vi "Test CD Mgr API.vi"() -> ()   [LabVIEW 2015]
doc: "Probe Mgr API Tester."
uses:
  Collect Data Mgr.lvlib
  Data Collect Parameters typedef--cluster.ctl
  Tool Module/Tool Module.lvlib
  Tool Config/Tool Cfg.lvlib
  Tool Interface/Tool Interface.lvlib
  Tool Interface/_Host - HS Data Stream State Enum Typedef.ctl
  Tool Typedefs/_Data Stream Fmt Params Cluster--typedef.ctl
  Start Collect (Reply Payload)--cluster.ctl
  Stop Collect (Reply Payload)--cluster.ctl
panel:
  in  "data value reference":refnum<data-value>
  out "All Stop":bool
  out "latest notification":u32[](array[numeric])
  out "Position Plot":i32[](graph)
  out "Fault":u8
  out "Position":i32
  in  "Move to Scan Start":bool
  out "Fault or Limit?":bool
  out "At Home?":bool
  in  "Check Home":bool
  in  "Home":bool
  out "Connected":bool
  out "Reply Payload":T1
  in  "Stop Collect":bool
  out "Start Collect (Reply Payload)":T2
  in  "Start Collect":bool
  in  "Show Block Diagram":bool
  in  "Stop Module":bool
  in  "Start Module":bool
  in  "Hide Module Panel":bool
  in  "Show Module Panel":bool
  out "Status":string
  out "Module Running?":bool
  # "This VI tests the API for the Module."
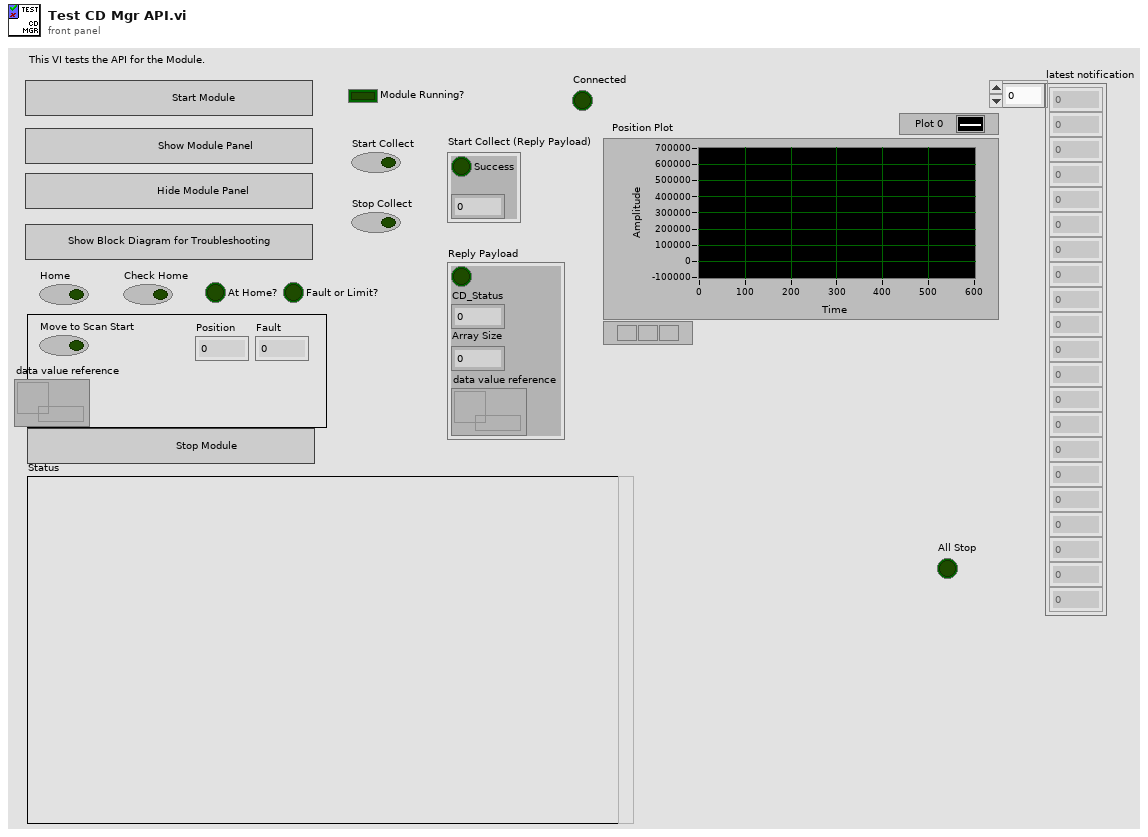
[diagram p1: front panel]
types:
  T1 = typedef "Collect Data Mgr.lvlib/Stop Collect (Reply Payload)--cluster.ctl" = cluster{"Success":bool, "CD_Status":i32, "Array Size":u32, "data value reference":refnum<data-value>}
  T2 = typedef "Collect Data Mgr.lvlib/Start Collect (Reply Payload)--cluster.ctl" = cluster{"Success":bool, "CD_Status":u8}
  T3 = typedef "Tool Interface.lvlib/_Host - HS Data Stream State Enum Typedef.ctl" = enum16{"Idle", "Connect", "Receive Data", "Close Connection"}
  T4 = typedef "Tool Interface.lvlib/_Host - HS Data Stream State Enum Typedef.ctl" = enum16{"Idle", "Connect", "Receive HS Data", "Close Connection"}
  T5 = typedef "Tool Cfg.lvlib/_Tool Operation Config Cluster--typedef.ctl" = cluster{"Use Tool Cfg":bool, "Use Tool Cal":bool, "Fake Data?":bool, "Mode":i16, "Array Subset Length":i16, "nArrays to Read":i16, "Full Array Read Length":i16, "nSubarrays/Sensor":i16}
  T6 = typedef "Collect Data Mgr.lvlib/Broadcast Events--cluster.ctl" = cluster{"Module Did Init":refnum<user-event>, "Status Updated":refnum<user-event>, "Error Reported":refnum<user-event>, "Module Did Stop":refnum<user-event>, "Update Module Execution Status":refnum<user-event>}
  T7 = typedef "_Data Stream Fmt Params Cluster--typedef.ctl" = cluster{"Samples per Block":i32, "Raw Data Status Len":i32, "Fltr Data Status Len":i32}
  T8 = typedef "Collect Data Mgr.lvlib/Data Collect Parameters typedef--cluster.ctl" = cluster{"Mode":i8, "Move Length":i32, "Array Length":i32, "Max Samples":i32}
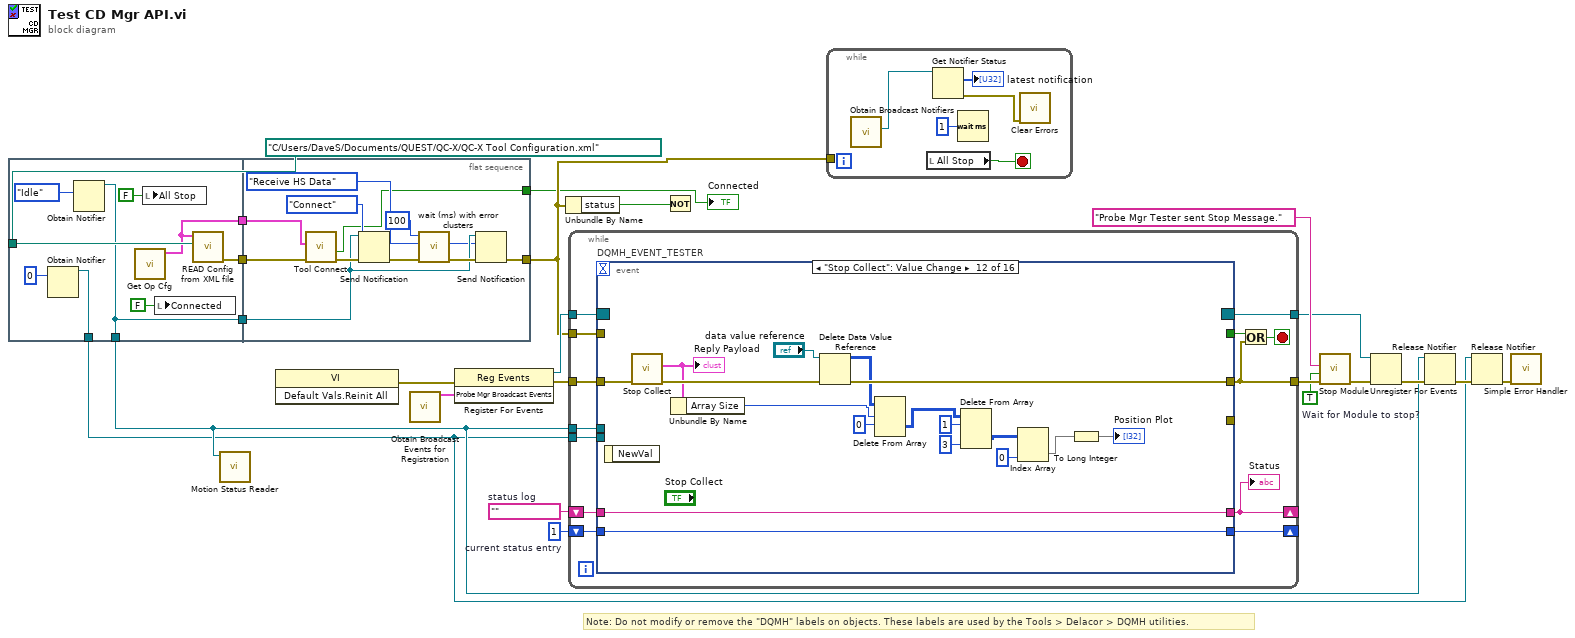
[diagram p0: block diagram]
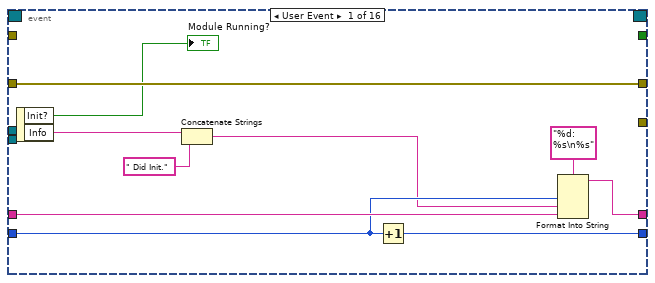
[diagram p2: hidden frame]
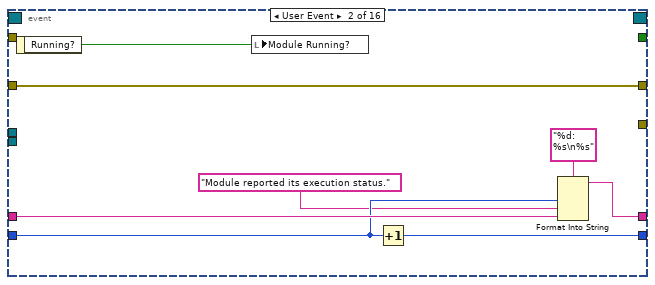
[diagram p3: hidden frame]
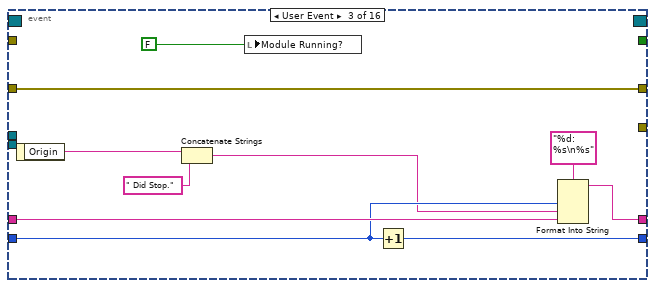
[diagram p4: hidden frame]
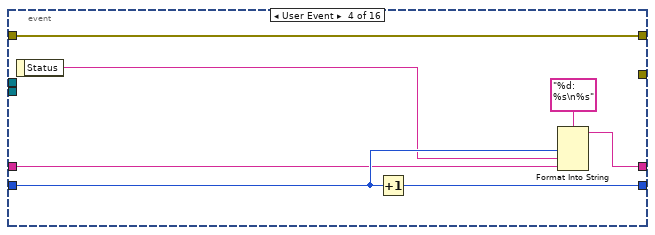
[diagram p5: hidden frame]
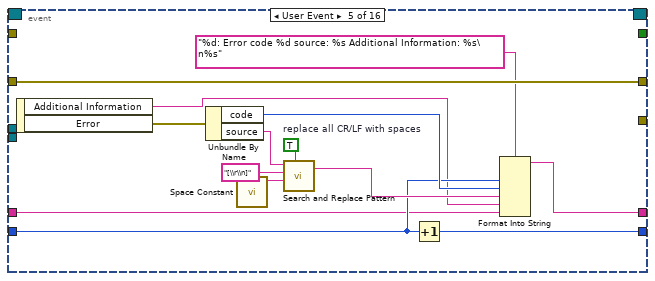
[diagram p6: hidden frame]
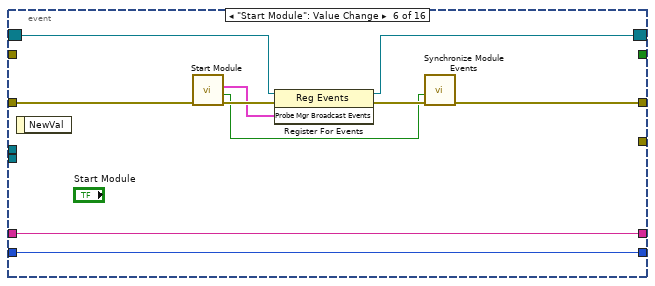
[diagram p7: hidden frame]
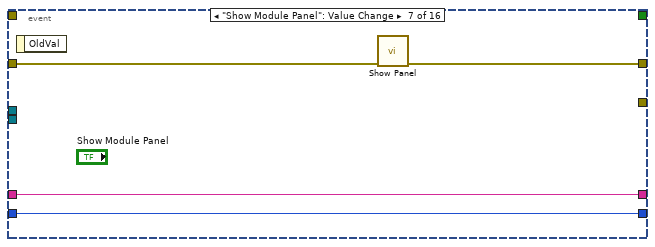
[diagram p8: hidden frame]
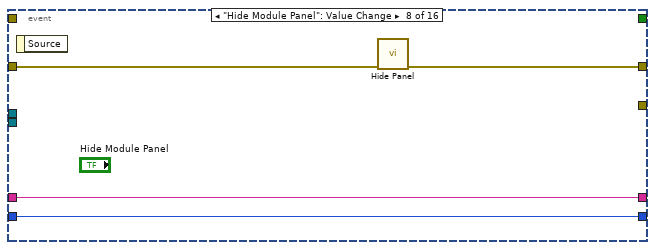
[diagram p9: hidden frame]
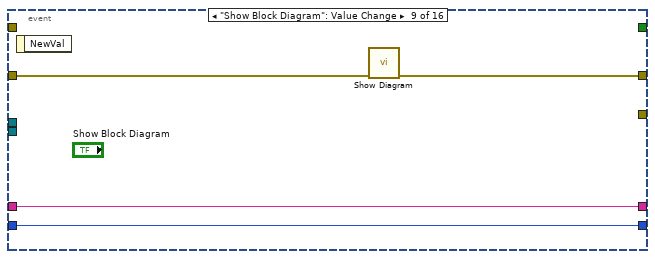
[diagram p10: hidden frame]
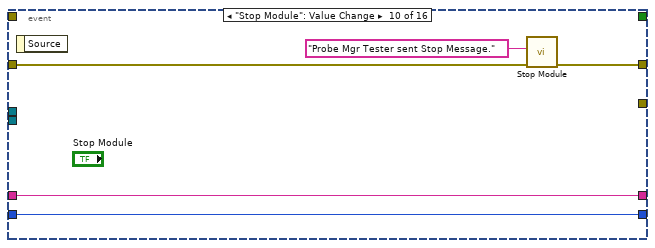
[diagram p11: hidden frame]
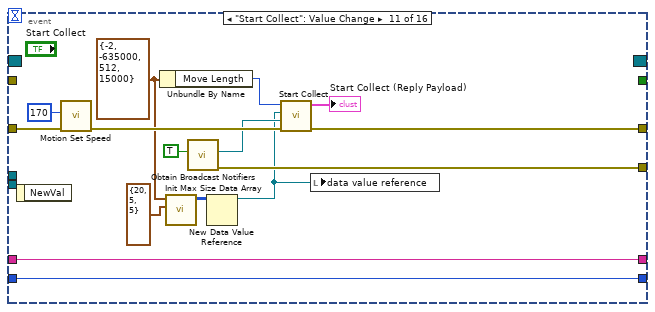
[diagram p12: hidden frame]
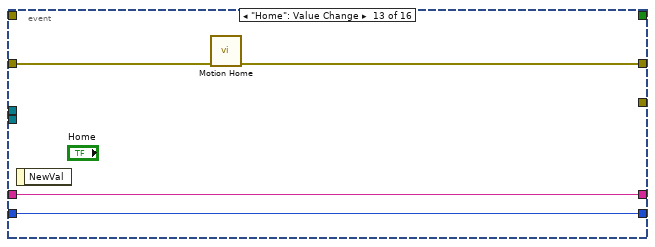
[diagram p13: hidden frame]
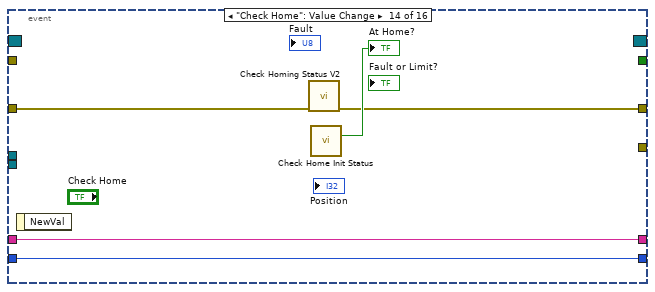
[diagram p14: hidden frame]
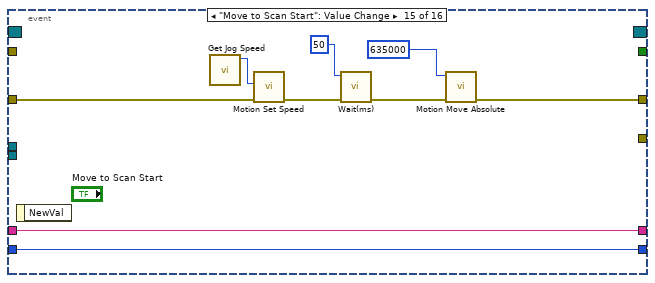
[diagram p15: hidden frame]
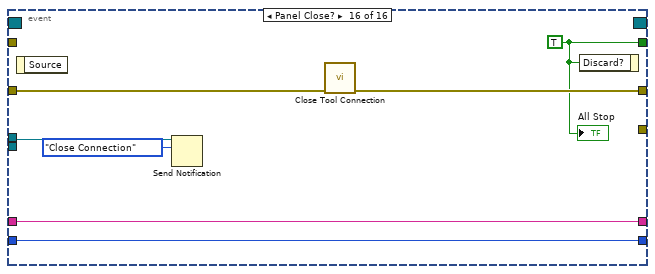
[diagram p16: hidden frame]
diagram:
  w13 = TRUE  # Wait for Module to stop?
  w19 = 1  # current status entry
  w20 = ""  # status log
  # "Note: Do not modify or remove the \"DQMH\" labels on objects. These labels are used by the Tools > Delacor > DQMH utilities."
  n1 = flat-sequence {
    tunnel: [w30] -> w12
    tunnel: path "C:/Users/DaveS/Documents/QUEST/QC-X/QC-X Tool Configuration.xml" -> [w31]
    tunnel: [w29] -> w9
    tunnel: [w27] -> w7
    tunnel: [w27] -> w5
    tunnel: [w24] -> w2
    tunnel: [w38] -> w6
    tunnel: w12 -> [w41]
    tunnel: w9 -> [w42]
    tunnel: w7 -> [w36]
    tunnel: [w33] -> w1
    frame #0 {
      n2 = Obtain Notifier(notification data type=u32 0) -> (notifier out=w24:refnum<notifier>)  [unwired: 3 in, 2 out]
      n3 = Obtain Notifier(notification data type=_Host_-_HS_Data_Stream_State_Enum_Typedef."Idle" ("RT Loop - HS Data Stream State Typedef")) -> (notifier out=w27:refnum<notifier>)  [unwired: 3 in, 2 out]
      n4 = call "Get Op Cfg.vi"() -> ("Tool Operation Config"=w29:T5)  [unwired: 11 in]
      n5 = local write "All Stop"(FALSE ("All Stop")) -> ()
      n6 = local write "Connected"(FALSE ("Connected")) -> ()
      n7 = call "READ Config from XML file.vi"("Path"=w31, "Default Op Config"=w29) -> ("error out"=w30:errorcluster)  [unwired: 6 in, 3 out]
    }
    frame #1 {
      n8 = call "Tool Connect.vi"("error in (no error)"=w41, "Tool Operation Config"=w42) -> ("Connected"=w33:bool)  [unwired: 4 in, 5 out]
      n9 = Send Notification(notification=_Host_-_HS_Data_Stream_State_Enum_Typedef."Connect", notifier=w36, error in (no error)=w41) -> (error out=w40:errorcluster)  [unwired: 1 out]
      n10 = call "wait (ms) with error clusters.vi"("error in (no error)"=w40, "milliseconds to wait"=u32 100) -> ("error out"=w39:errorcluster)  [unwired: 9 in]
      n11 = Send Notification(notification=_Host_-_HS_Data_Stream_State_Enum_Typedef."Receive HS Data", notifier=w36, error in (no error)=w39) -> (error out=w38:errorcluster)  [unwired: 1 out]
    }
  }
  n12 = call "Motion Status Reader.vi"("Control"=w5) -> ()  [unwired: 11 in]
  n13 = invoke class="VI" method="Default Vals.Reinit All"() -> (error out=w18:errorcluster)  [unwired: 3 in, 2 out]
  n14 = call "Obtain Broadcast Events for Registration.vi"() -> ("Probe Mgr Broadcast Events"=w16:T6)  [unwired: 9 in, 2 out]
  n15 = register-events(error in=w18, w16) -> (reference out=w15:refnum<event-registration>, error out=w17:errorcluster)  [unwired: 1 in]
  n16 = Unbundle By Name(w6) -> ("status"=w10:bool)
  n17 = while {
    tunnel: w15 -> [w55]
    tunnel: [w48] -> w22
    shift-right: [w50] -> _
    shift-left: w20 -> [w52]
    shift-right: [w51] -> _
    shift-left: w19 -> [w53]
    tunnel: w17 -> [w47]
    tunnel: [w46] -> w14
    tunnel: w6 -> [w45]
    tunnel: w5 -> [w44]
    tunnel: w2 -> [w43]
    stop <- w49 stop-if-true
    n18 = event "DQMH_EVENT_TESTER" shown="[11] \"Stop Collect\": Value Change" {
      selector: w55 -> [_ _ _ _ _ w108 _ _ _ _ _ _ _ _ _ _]
      dyn-events: [_ _ _ _ _ w107 _ _ _ _ _ _ _ _ _ _] -> w46
      timeout: _ -> [_ _ _ _ _ _ _ _ _ _ _ _ _ _ _ _]
      tunnel: [_ _ _ _ _ _ _ _ _ _ _ _ _ _ _ w182] -> w54
      tunnel: [w65 w67 w74 w84 w104 w106 w118 w122 w123 w129 w141 w163 w164 w169 w173 w186] -> w48
      tunnel: w53 -> [w61 w71 w81 w87 w94 w111 w116 w120 w124 w130 w144 w161 w166 w171 w180 w187]
      tunnel: w52 -> [w62 w72 w82 w86 w92 w112 w117 w121 w125 w131 w145 w162 w167 w172 w181 w188]
      tunnel: [w59 w69 w79 w88 w95 w112 w117 w121 w125 w131 w145 w162 w167 w172 w181 w188] -> w50
      tunnel: [w60 w70 w80 w90 w93 w111 w116 w120 w124 w130 w144 w161 w166 w171 w180 w187] -> w51
      tunnel: w47 -> [w65 w67 w74 w84 w104 w105 w115 w119 w126 w127 w138 w160 w165 w168 w179 w183]
      tunnel: w45 -> [_ _ _ _ _ _ _ _ _ _ _ _ _ _ _ _]
      tunnel: [_ _ _ _ _ _ _ _ _ _ w139 _ _ _ _ _] -> _
      tunnel: w44 -> [_ _ _ _ _ _ _ _ _ _ _ _ _ _ _ w185]
      tunnel: w43 -> [_ _ _ _ _ _ _ _ _ _ _ _ _ _ _ _]
      event User Event {
        n19 = event-data() -> ("Init?"=→"Module Running?":bool, "Info"=w58:string)  [unwired: 1 in]
        n20 = Concatenate Strings(w58, " Did Init.") -> (w57:string)
        n21 = Increment(x=w61) -> (x+1=w60:i32)
        n22 = Format Into String(format string="%d: %s\n%s", w61, w57, w62) -> (resulting string=w59:string)  [unwired: 2 in, 1 out]
      }
      event User Event {
        n23 = event-data() -> ("Running?"=w66:bool)  [unwired: 1 in]
        n24 = local write "Module Running?"(w66) -> ()
        n25 = Increment(x=w71) -> (x+1=w70:i32)
        n26 = Format Into String(format string="%d: %s\n%s", w71, "Module reported its execution status.", w72) -> (resulting string=w69:string)  [unwired: 2 in, 1 out]
      }
      event User Event {
        n27 = event-data() -> ("Origin"=w78:string)  [unwired: 1 in]
        n28 = Concatenate Strings(w78, " Did Stop.") -> (w77:string)
        n29 = local write "Module Running?"(FALSE ("Module Did Init?")) -> ()
        n30 = Increment(x=w81) -> (x+1=w80:i32)
        n31 = Format Into String(format string="%d: %s\n%s", w81, w77, w82) -> (resulting string=w79:string)  [unwired: 2 in, 1 out]
      }
      event User Event {
        n32 = event-data() -> ("Status"=w85:string)  [unwired: 1 in]
        n33 = Increment(x=w87) -> (x+1=w90:i32)
        n34 = Format Into String(format string="%d: %s\n%s", w87, w85, w86) -> (resulting string=w88:string)  [unwired: 2 in, 1 out]
      }
      event User Event {
        w100 = TRUE  # replace all CR/LF with spaces
        n35 = event-data() -> ("Additional Information"=w91:string, "Error"=w96:errorcluster)  [unwired: 1 in]
        n36 = Unbundle By Name(w96) -> ("code"=w97:i32, "source"=w98:string)
        n37 = call <vilib>:"Space Constant.vi"() -> ("String"=w101:string)
        n38 = call <vilib>:"Search and Replace Pattern.vi"("string"=w98, "regular expression (\"\")"="[\\r\\n]" ("regular expression (\"\")"), "replace string (\"\")"=w101, "replace all? (F)"=w100) -> ("result string"=w99:string)  [unwired: 1 in, 1 out]
        n39 = Increment(x=w94) -> (x+1=w93:i32)
        n40 = Format Into String(format string="%d: Error code %d source: %s Additional Information: %s\n%s", w94, w97, w99, w91, w92) -> (resulting string=w95:string)  [unwired: 2 in, 1 out]
      }
      event "Start Module": Value Change {
        n41 = event-data() -> ()  [unwired: 1 in, 1 out]
        n42 = call "Start Module.vi"("error in (no error)"=w105) -> ("error out"=w113:errorcluster, "Wait for Event Sync?"=w110:bool, "Probe Mgr Broadcast Events"=w109:T6)  [unwired: 8 in]
        n43 = register-events(reference=w108, error in=w113, w109) -> (reference out=w107:refnum<event-registration>, error out=w114:errorcluster)
        n44 = call "Synchronize Module Events.vi"("error in (no error)"=w114, "Wait for Event Sync?"=w110) -> ("error out"=w106:errorcluster)  [unwired: 9 in]
      }
      event "Show Module Panel": Value Change {
        n45 = event-data() -> ()  [unwired: 1 in, 1 out]
        n46 = call "Show Panel.vi"("error in (no error)"=w115) -> ("error out"=w118:errorcluster)  [unwired: 10 in]
      }
      event "Hide Module Panel": Value Change {
        n47 = event-data() -> ()  [unwired: 1 in, 1 out]
        n48 = call "Hide Panel.vi"("error in (no error)"=w119) -> ("error out"=w122:errorcluster)  [unwired: 10 in]
      }
      event "Show Block Diagram": Value Change {
        n49 = event-data() -> ()  [unwired: 1 in, 1 out]
        n50 = call "Show Diagram.vi"("error in (no error)"=w126) -> ("error out"=w123:errorcluster)  [unwired: 10 in]
      }
      event "Stop Module": Value Change {
        n51 = event-data() -> ()  [unwired: 1 in, 1 out]
        n52 = call "Stop Module.vi"("error in (no error)"=w127, "Origin"="Probe Mgr Tester sent Stop Message.") -> ("error out"=w129:errorcluster)  [unwired: 9 in]
      }
      event "Start Collect": Value Change {
        w133 = T8 {"Mode"=-2, "Move Length"=-635000, "Array Length"=512, "Max Samples"=15000} ("Data Collect Params")
        n53 = event-data() -> ()  [unwired: 1 in, 1 out]
        n54 = call "Motion Set Speed.vi"("error in (no error)"=w138, "Speed"=u16 170) -> ("error out"=w146:errorcluster)  [unwired: 9 in]
        n55 = Unbundle By Name(w133) -> ("Move Length"=w132:i32)
        n56 = call "Init Max Size Data Array.vi"("Data Stream Fmt Params"=T7 {"Samples per Block"=20, "Raw Data Status Len"=5, "Fltr Data Status Len"=5} ("Acq  Process Params"), "Data Collect Params"=w133) -> ("initialized array"=w135:u32[][])  [unwired: 9 in]
        n57 = call "Obtain Broadcast Notifiers.vi"("Create New?"=TRUE) -> ("error out"=w139:errorcluster, "Sample Data notifier out"=w143:refnum<notifier>)  [unwired: 9 in]
        n58 = New Data Value Reference(data value=w135) -> (data value reference=w134:refnum<data-value>)  [unwired: 1 in, 1 out]
        n59 = call "Start Collect.vi"("error in (no error)"=w146, "Sample Data notifier"=w143, "data value reference"=w134, "Move Length"=w132) -> ("error out"=w141:errorcluster, "Start Collect (Reply Payload)"=→"Start Collect (Reply Payload)":T2)  [unwired: 5 in, 1 out]
        n60 = local write "data value reference"(w134) -> ()
      }
      event "Stop Collect": Value Change {
        n61 = event-data() -> ()  [unwired: 1 in, 1 out]
        n62 = call "Stop Collect.vi"("error in (no error)"=w160) -> ("error out"=w152:errorcluster, "Reply Payload"=w151:T1)  [unwired: 8 in, 1 out]
        "Reply Payload" <- w151
        n63 = Unbundle By Name(w151) -> ("Array Size"=w148:u32)
        n64 = Delete Data Value Reference(data value reference="data value reference", error in=w152) -> (data value=w150:u32[][], error out=w163:errorcluster)
        n65 = Delete From Array(array=w150, length=w148, index (row)=0) -> (deleted portion=w147:u32[][])  [unwired: 1 in, 1 out]
        n66 = Delete From Array(array=w147, length=1, index (col)=3 ("disabled index (col)")) -> (deleted portion=w157:u32[][])  [unwired: 1 in, 1 out]
        n67 = Index Array(array=w157, index (col)=0 ("disabled index (col)")) -> (element=w156:u32[])  [unwired: 1 in]
        n68 = To Long Integer(number=w156) -> (32bit integer=→"Position Plot":i32[])
      }
      event "Home": Value Change {
        n69 = event-data() -> ()  [unwired: 1 in, 1 out]
        n70 = call "Motion Home.vi"("error in (no error)"=w165) -> ("error out"=w164:errorcluster)  [unwired: 10 in]
      }
      event "Check Home": Value Change {
        n71 = event-data() -> ()  [unwired: 1 in, 1 out]
        n72 = call "Check Homing Status V2.vi"("error in (no error)"=w168) -> ("error out"=w169:errorcluster)  [unwired: 8 in, 2 out]
        n73 = call "Check Home Init Status.vi"() -> ("Home Init?"=→"At Home?":bool)  [unwired: 15 in]
      }
      event "Move to Scan Start": Value Change {
        n74 = event-data() -> ()  [unwired: 1 in, 1 out]
        n75 = call "Get Jog Speed.vi"() -> ("Jog Speed"=w178:u16)  [unwired: 11 in]
        n76 = call "Motion Set Speed.vi"("error in (no error)"=w179, "Speed"=w178) -> ("error out"=w177:errorcluster)  [unwired: 9 in]
        n77 = call "Wait(ms).vi"("error in (no error)"=w177, "milliseconds"=u32 50 ("Milliseconds to wait")) -> ("error out"=w174:errorcluster)  [unwired: 9 in]
        n78 = call "Motion Move Absolute.vi"("error in (no error)"=w174, "Position"=635000 ("jog increment")) -> ("error out"=w173:errorcluster)  [unwired: 9 in]
      }
      event Panel Close? {
        w182 = TRUE ("Discard?")
        n79 = event-data() -> ()  [unwired: 1 in, 1 out]
        n80 = Send Notification(notification=_Host_-_HS_Data_Stream_State_Enum_Typedef."Close Connection", notifier=w185) -> ()  [unwired: 1 in, 2 out]
        n81 = call "Close Tool Connection.vi"("error in (no error)"=w183) -> ("error out"=w186:errorcluster)  [unwired: 10 in]
        n82 = event-data("Discard?"=w182) -> ()  [unwired: 1 in, 1 out]
        "All Stop" <- w182
      }
    }
    "Status" <- w50
    n83 = Or(x=w54, y=w48) -> (x .or. y?=w49:bool)
  }
  n84 = Not(x=w10) -> ()  [unwired: 1 out]
  n85 = while {
    tunnel: w6 -> [_]
    stop <- w193 stop-if-true
    n86 = call "Obtain Broadcast Notifiers.vi"() -> ("Sample Data notifier out"=w191:refnum<notifier>)  [unwired: 10 in, 1 out]
    n87 = local read "All Stop"() -> (w193:bool)
    n88 = Get Notifier Status(notifier=w191) -> (current notification=→"latest notification":u32[], error out=w190:errorcluster)  [unwired: 1 in, 3 out]
    n89 = Wait (ms)(milliseconds to wait=u32 1) -> ()  [unwired: 1 out]
    n90 = call <vilib>:"Clear Errors.vi"("error in (no error)"=w190) -> ()  [unwired: 5 in, 2 out]
  }
  n91 = call "Stop Module.vi"("error in (no error)"=w22, "Wait for Module to Stop? (F)"=w13, "Origin"="Probe Mgr Tester sent Stop Message.") -> ("error out"=w23:errorcluster)  [unwired: 8 in]
  n92 = Unregister For Events(event registration refnum=w14, error in=w23) -> (error out=w8:errorcluster)
  n93 = Release Notifier(notifier=w5, error in (no error)=w8) -> (error out=w4:errorcluster)  [unwired: 1 in, 2 out]
  n94 = Release Notifier(notifier=w2, error in (no error)=w4) -> (error out=w3:errorcluster)  [unwired: 1 in, 2 out]
  n95 = call <vilib>:"Simple Error Handler.vi"("error in (no error)"=w3) -> ()  [unwired: 4 in, 5 out]
  "Connected" <- w1
